vi "gds_receiver.vi"(8 "error in (no error)":errorcluster, 9 "Received Bit Sequence":i8[](array[numeric]) caption="Key Bit Sequence", 10 "Received Signal":T3={"t0"=0.0, "dt"=1.0, "Y"=[]} {"Y" format="%.3f"; "dt" format="%^.2e"; "t0" format="%.4f"}, 11 "Modulation Parameters":T1) -> (0 "error out":errorcluster, 1 "Measurements":T2 caption="measurements" {"FSK error (Hz)" format="%.2f"; "deviation error (Hz)" format="%.2f"; "frequency drift (Hz)" format="%.2f"; "frequency offset (Hz)" format="%.2f"}, 2 "BER":dbl, 3 "Key Bit Sequence":i8[](array[numeric]) caption="Recovered Bit Sequence", 4 "recovered complex waveform":T3 {"Y" format="%.3f"; "dt" format="%^.2e"; "t0" format="%.4f"})   [LabVIEW 2012]
uses:
  <vilib>/addons/Modulation/Analog/controls/Complex Data Waveform.ctl
  <vilib>/addons/Modulation/niAMT.lvlib
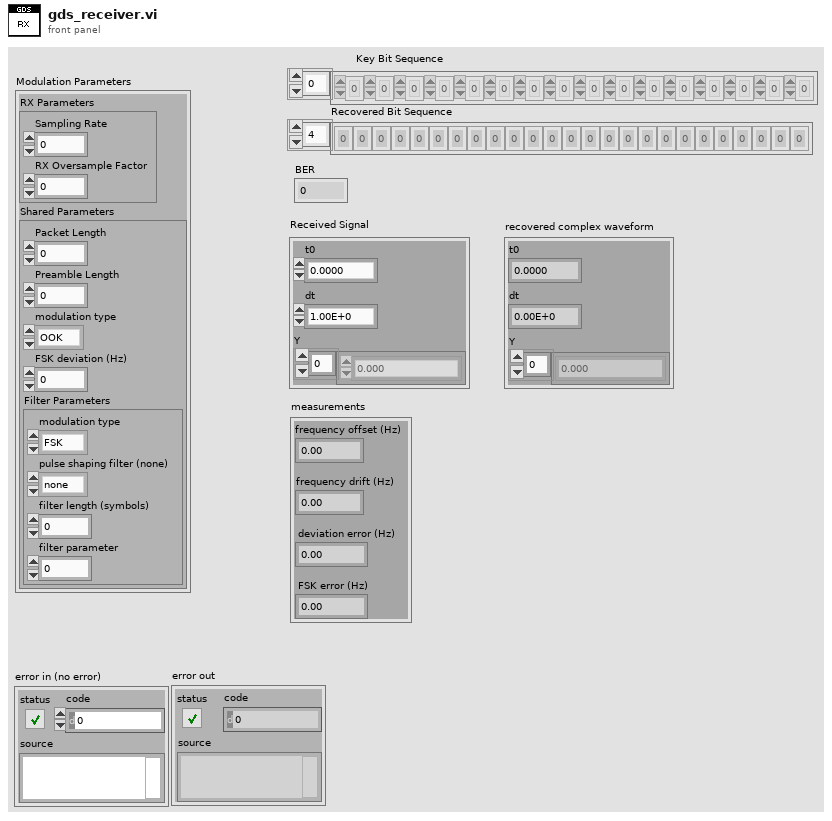
[diagram p1: front panel]
types:
  T1 = cluster{"RX Parameters":cluster{"Sampling Rate":dbl, "RX Oversample Factor":i32}, "Shared Parameters":cluster{"Packet Length":i32, "Preamble Length":i32, "modulation type":enum16{"OOK", "FSK", "PSK", "QAM", "MSK", "PAM", "ASK", "CPM"}, "FSK deviation (Hz)":dbl, "Filter Parameters":cluster{"modulation type":enum16{"FSK", "PSK", "QAM", "MSK", "PAM", "ASK", "CPM"}, "pulse shaping filter (none)":enum16{"none", "Raised Cosine", "Root Raised Cos", "Gaussian"}, "filter length (symbols)":i32, "filter parameter":dbl}}}
  T2 = cluster{"frequency offset (Hz)":dbl, "frequency drift (Hz)":dbl, "deviation error (Hz)":dbl, "FSK error (Hz)":dbl}
  T3 = typedef "niAMT.lvlib/Complex Data Waveform.ctl" = cluster{"t0":dbl, "dt":dbl, "Y":cdb[]}
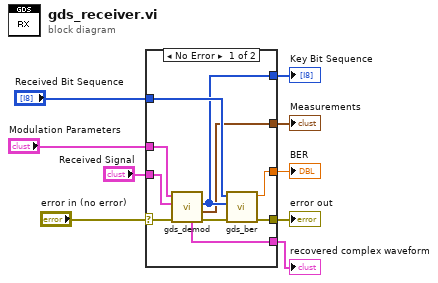
[diagram p0: block diagram]
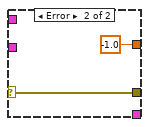
[diagram p2: hidden frame]
diagram:
  n1 = case shown="No Error" "error in (no error)" {
    selector: "error in (no error)" -> [w16 w21]
    tunnel: [w19 w21] -> w8
    tunnel: "Received Bit Sequence" -> [w18 _]
    tunnel: [w14 _] -> w6
    tunnel: [w17 -1.0 ("BER")] -> w5
    tunnel: "Received Signal" -> [w13 _]
    tunnel: "Modulation Parameters" -> [w12 _]
    tunnel: [w11 _] -> w2
    tunnel: [w10 _] -> w1
    frame No Error {
      n2 = call "gds_demod.vi"("error in (no error)"=w16, "input complex waveform"=w13, "Modulation Parameters"=w12) -> ("error out"=w15:errorcluster, "Measurements"=w11:T2, "output bit stream"=w14:i8[], "recovered complex waveform"=w10:T3)  [unwired: 4 in, 1 out]
      n3 = call "gds_ber.vi"("error in (no error)"=w15, "Recovered Bit Sequence"=w14, "Received Bit Sequence"=w18) -> ("error out"=w19:errorcluster, "BER"=w17:dbl)  [unwired: 7 in]
    }
    frame Error {
    }
  }
  "Key Bit Sequence" <- w6
  "error out" <- w8
  "BER" <- w5
  "recovered complex waveform" <- w1
  "Measurements" <- w2
